vi "83-86 (SubVI).vi"(1 "String":string) -> (0 "Output":T1)   [LabVIEW 2024]
panel:
  in  "Output 2":T1
  in  "Carrier Card Temperature alert 2":T2
  in  "Switching Card 5 Temperature alert 2":T3
  in  "Switching Card 4 Temperature alert 2":T4
  in  "Switching Card 3 Temperature alert 2":T5
  in  "Switching Card 2 Temperature alert 2":T6
  in  "Switching Card 1 Temperature alert  2":T7
  in  "Control Card Temperature alert  2":T8
  in  "Carrier Card Temperature Warning 2":T9
  in  "Switching Card 5 Temperature Warning 2":T10
  in  "Switching Card 4 Temperature  Warning 2":T11
  in  "Switching Card 3 Temperature Warning 2":T12
  in  "Switching Card 2 Temperature High Warning 2":T13
  in  "Switching Card 1 Temperature Warning 2":T14
  in  "Control Card Temperature Warning 2":T15
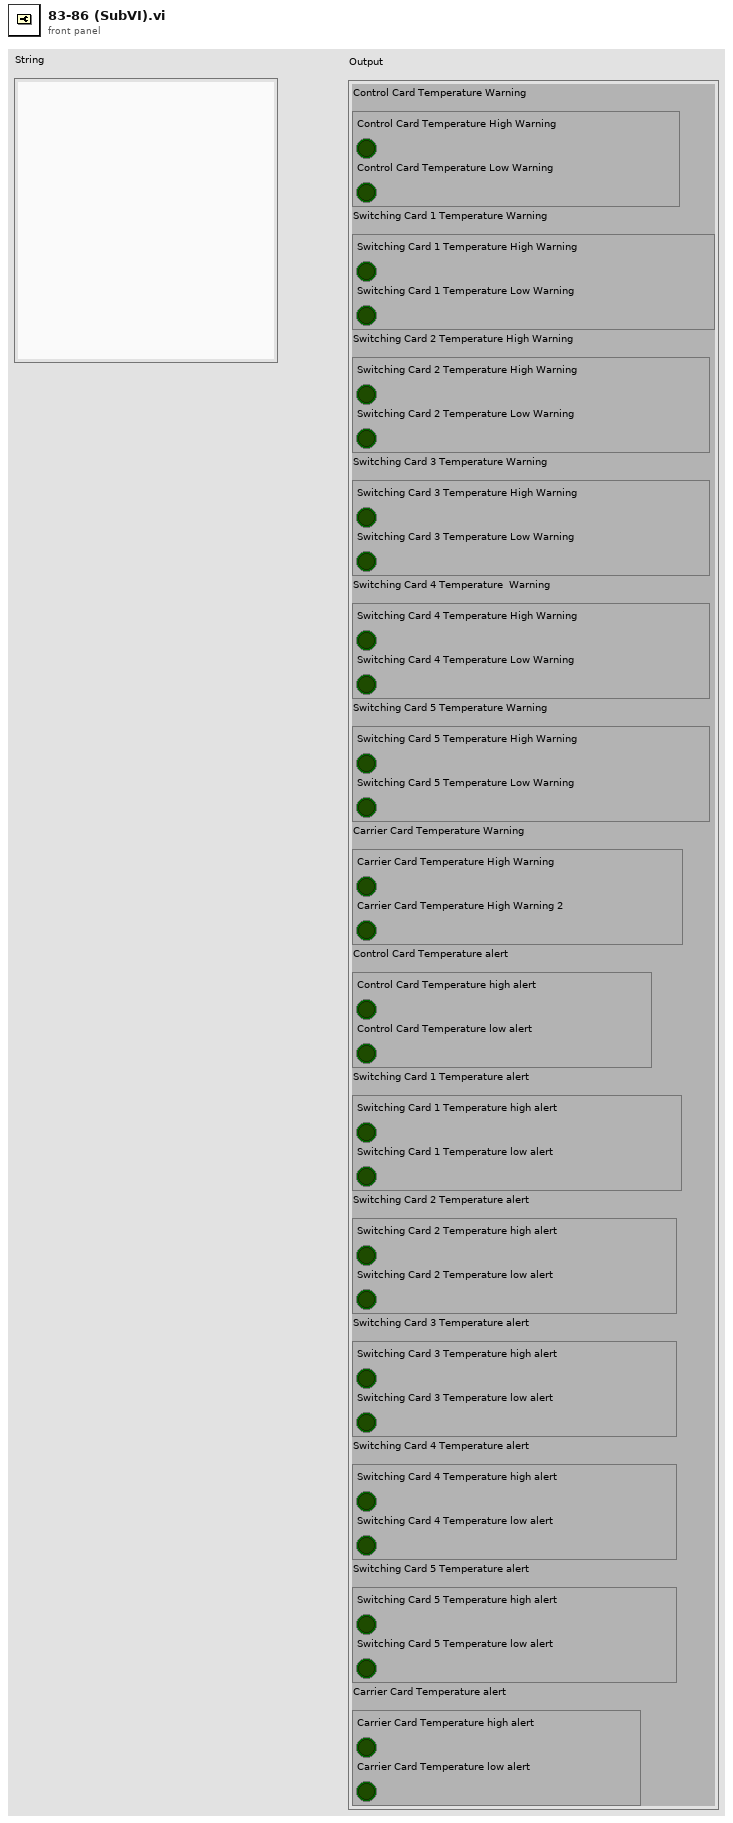
[diagram p1: front panel]
types:
  T1 = cluster{"Control Card Temperature Warning":cluster{"Control Card Temperature High Warning ":bool, "Control Card Temperature Low Warning":bool}, "Switching Card 1 Temperature Warning":cluster{"Switching Card 1 Temperature High Warning ":bool, "Switching Card 1 Temperature Low Warning":bool}, "Switching Card 2 Temperature High Warning":cluster{"Switching Card 2 Temperature High Warning":bool, "Switching Card 2 Temperature Low Warning":bool}, "Switching Card 3 Temperature Warning":cluster{"Switching Card 3 Temperature High Warning":bool, "Switching Card 3 Temperature Low Warning":bool}, "Switching Card 4 Temperature  Warning":cluster{"Switching Card 4 Temperature High Warning":bool, "Switching Card 4 Temperature Low Warning":bool}, "Switching Card 5 Temperature Warning":cluster{"Switching Card 5 Temperature High Warning":bool, "Switching Card 5 Temperature Low Warning":bool}, "Carrier Card Temperature Warning":cluster{"Carrier Card Temperature High Warning":bool, "Carrier Card Temperature High Warning 2":bool}, "Control Card Temperature alert ":cluster{"Control Card Temperature high alert ":bool, "Control Card Temperature low alert ":bool}, "Switching Card 1 Temperature alert ":cluster{"Switching Card 1 Temperature high alert ":bool, "Switching Card 1 Temperature low alert ":bool}, "Switching Card 2 Temperature alert":cluster{"Switching Card 2 Temperature high alert":bool, "Switching Card 2 Temperature low alert":bool}, "Switching Card 3 Temperature alert":cluster{"Switching Card 3 Temperature high alert":bool, "Switching Card 3 Temperature low alert":bool}, "Switching Card 4 Temperature alert":cluster{"Switching Card 4 Temperature high alert":bool, "Switching Card 4 Temperature low alert":bool}, "Switching Card 5 Temperature alert":cluster{"Switching Card 5 Temperature high alert":bool, "Switching Card 5 Temperature low alert":bool}, "Carrier Card Temperature alert":cluster{"Carrier Card Temperature high alert":bool, "Carrier Card Temperature low alert":bool}}
  T2 = cluster{"Carrier Card Temperature high alert":bool, "Carrier Card Temperature low alert":bool}
  T3 = cluster{"Switching Card 5 Temperature high alert":bool, "Switching Card 5 Temperature low alert":bool}
  T4 = cluster{"Switching Card 4 Temperature high alert":bool, "Switching Card 4 Temperature low alert":bool}
  T5 = cluster{"Switching Card 3 Temperature high alert":bool, "Switching Card 3 Temperature low alert":bool}
  T6 = cluster{"Switching Card 2 Temperature high alert":bool, "Switching Card 2 Temperature low alert":bool}
  T7 = cluster{"Switching Card 1 Temperature high alert ":bool, "Switching Card 1 Temperature low alert ":bool}
  T8 = cluster{"Control Card Temperature high alert ":bool, "Control Card Temperature low alert ":bool}
  T9 = cluster{"Carrier Card Temperature High Warning":bool, "Carrier Card Temperature High Warning 2":bool}
  T10 = cluster{"Switching Card 5 Temperature High Warning":bool, "Switching Card 5 Temperature Low Warning":bool}
  T11 = cluster{"Switching Card 4 Temperature High Warning":bool, "Switching Card 4 Temperature Low Warning":bool}
  T12 = cluster{"Switching Card 3 Temperature High Warning":bool, "Switching Card 3 Temperature Low Warning":bool}
  T13 = cluster{"Switching Card 2 Temperature High Warning":bool, "Switching Card 2 Temperature Low Warning":bool}
  T14 = cluster{"Switching Card 1 Temperature High Warning ":bool, "Switching Card 1 Temperature Low Warning":bool}
  T15 = cluster{"Control Card Temperature High Warning ":bool, "Control Card Temperature Low Warning":bool}
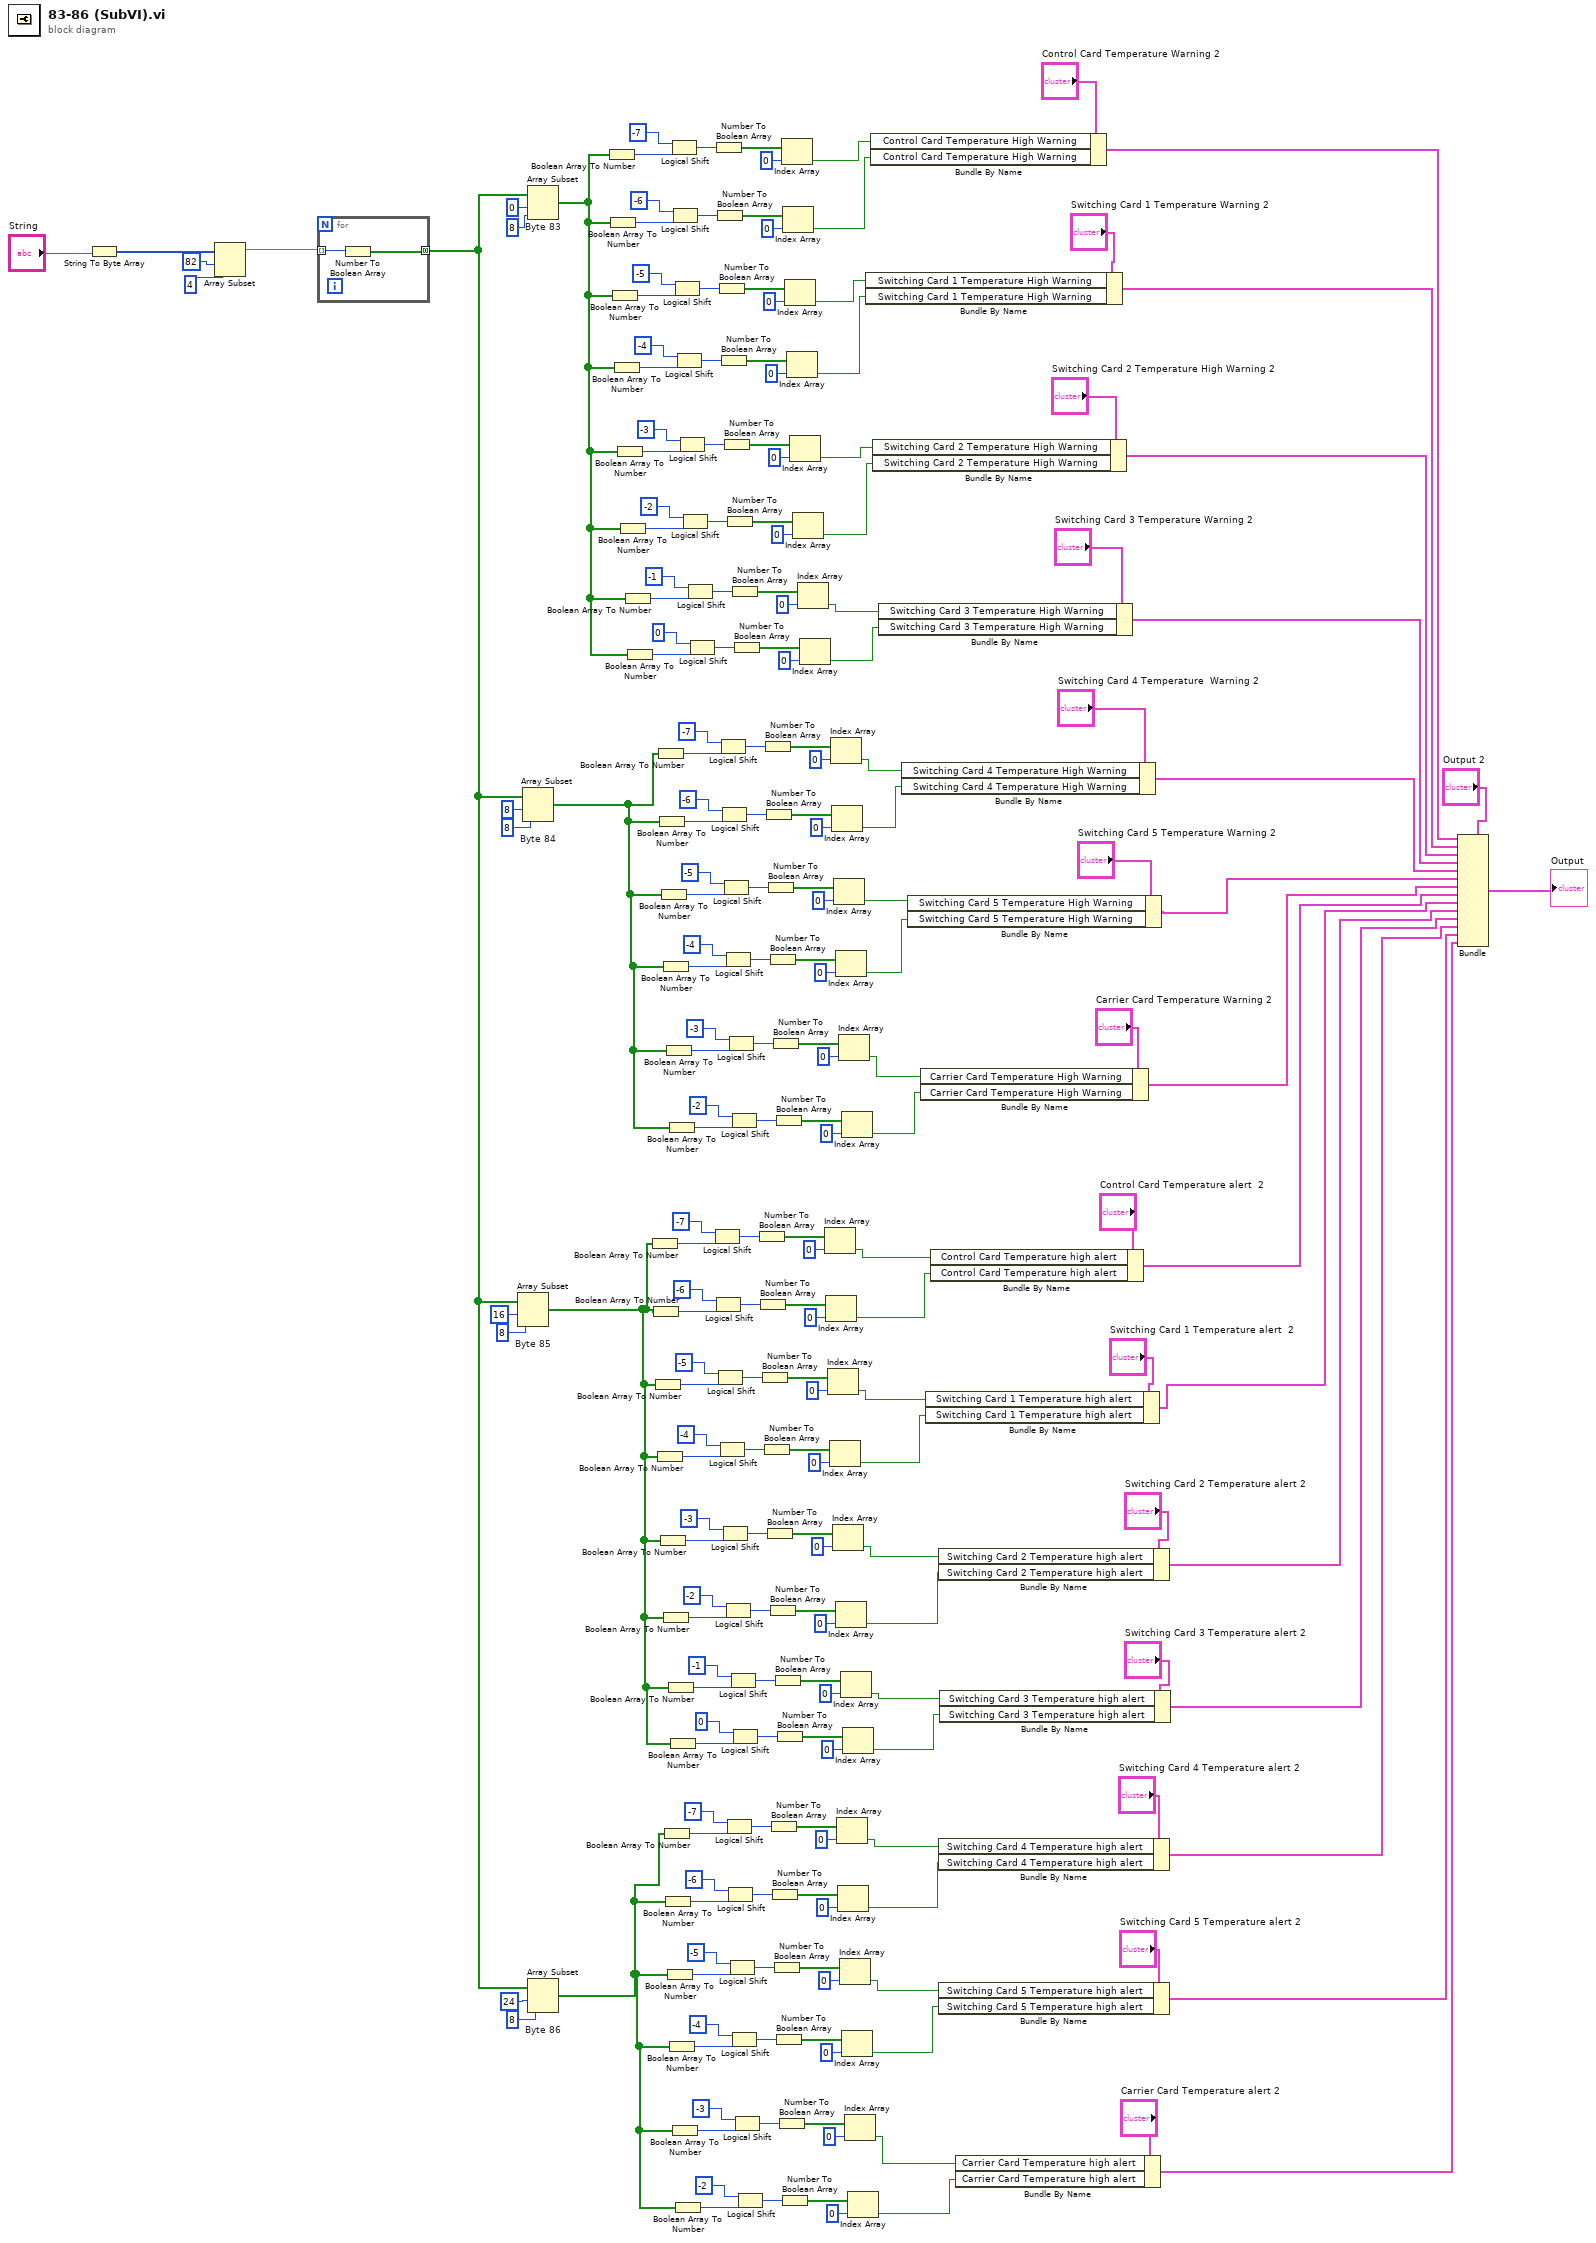
[diagram p0: block diagram]
diagram:
  n1 = String To Byte Array(string="String") -> (unsigned byte array=w209:u8[])
  n2 = Array Subset(array=w209, index=82, length=4) -> (w206:u8[])
  n3 = for {
    tunnel: w206 -> [w218] mode=indexing
    tunnel: [w217] -> w203 mode=concatenating
    n4 = Number To Boolean Array(number=w218) -> (Boolean array=w217:bool[])
  }
  n5 = Array Subset "Byte 85"(array=w203, index=16, length=8) -> (w90:bool[])
  n6 = Array Subset "Byte 84"(array=w203, index=8, length=8) -> (w131:bool[])
  n7 = Array Subset "Byte 83"(array=w203, index=0, length=8) -> (w162:bool[])
  n8 = Array Subset "Byte 86"(array=w203, index=24, length=8) -> (w59:bool[])
  n9 = Boolean Array To Number(Boolean array=w162) -> (number=w200:u32)
  n10 = Boolean Array To Number(Boolean array=w162) -> (number=w195:u32)
  n11 = Boolean Array To Number(Boolean array=w162) -> (number=w190:u32)
  n12 = Boolean Array To Number(Boolean array=w162) -> (number=w185:u32)
  n13 = Boolean Array To Number(Boolean array=w162) -> (number=w180:u32)
  n14 = Boolean Array To Number(Boolean array=w162) -> (number=w175:u32)
  n15 = Boolean Array To Number(Boolean array=w162) -> (number=w170:u32)
  n16 = Boolean Array To Number(Boolean array=w162) -> (number=w165:u32)
  n17 = Boolean Array To Number(Boolean array=w90) -> (number=w93:u32)
  n18 = Boolean Array To Number(Boolean array=w90) -> (number=w98:u32)
  n19 = Boolean Array To Number(Boolean array=w90) -> (number=w103:u32)
  n20 = Boolean Array To Number(Boolean array=w90) -> (number=w108:u32)
  n21 = Boolean Array To Number(Boolean array=w131) -> (number=w134:u32)
  n22 = Boolean Array To Number(Boolean array=w131) -> (number=w139:u32)
  n23 = Boolean Array To Number(Boolean array=w90) -> (number=w113:u32)
  n24 = Boolean Array To Number(Boolean array=w131) -> (number=w144:u32)
  n25 = Boolean Array To Number(Boolean array=w131) -> (number=w149:u32)
  n26 = Boolean Array To Number(Boolean array=w90) -> (number=w118:u32)
  n27 = Boolean Array To Number(Boolean array=w59) -> (number=w87:u32)
  n28 = Boolean Array To Number(Boolean array=w59) -> (number=w82:u32)
  n29 = Boolean Array To Number(Boolean array=w131) -> (number=w154:u32)
  n30 = Boolean Array To Number(Boolean array=w59) -> (number=w77:u32)
  n31 = Boolean Array To Number(Boolean array=w90) -> (number=w123:u32)
  n32 = Boolean Array To Number(Boolean array=w131) -> (number=w159:u32)
  n33 = Boolean Array To Number(Boolean array=w59) -> (number=w72:u32)
  n34 = Boolean Array To Number(Boolean array=w90) -> (number=w128:u32)
  n35 = Logical Shift(y=i16 -7, x=w200) -> (x << y=w202:u32)
  n36 = Logical Shift(y=i16 -6, x=w195) -> (x << y=w193:u32)
  n37 = Boolean Array To Number(Boolean array=w59) -> (number=w67:u32)
  n38 = Logical Shift(y=i16 -5, x=w190) -> (x << y=w192:u32)
  n39 = Boolean Array To Number(Boolean array=w59) -> (number=w62:u32)
  n40 = Logical Shift(y=i16 -4, x=w185) -> (x << y=w183:u32)
  n41 = Logical Shift(y=i16 -3, x=w180) -> (x << y=w182:u32)
  n42 = Logical Shift(y=i16 -2, x=w175) -> (x << y=w173:u32)
  n43 = Logical Shift(y=i16 -1, x=w170) -> (x << y=w172:u32)
  n44 = Logical Shift(y=i16 0, x=w165) -> (x << y=w163:u32)
  n45 = Logical Shift(y=i16 -7, x=w93) -> (x << y=w91:u32)
  n46 = Logical Shift(y=i16 -6, x=w98) -> (x << y=w100:u32)
  n47 = Number To Boolean Array(number=w202) -> (Boolean array=w199:bool[])
  n48 = Number To Boolean Array(number=w193) -> (Boolean array=w196:bool[])
  n49 = Logical Shift(y=i16 -5, x=w103) -> (x << y=w101:u32)
  n50 = Number To Boolean Array(number=w192) -> (Boolean array=w189:bool[])
  n51 = Logical Shift(y=i16 -4, x=w108) -> (x << y=w110:u32)
  n52 = Logical Shift(y=i16 -7, x=w134) -> (x << y=w132:u32)
  n53 = Number To Boolean Array(number=w183) -> (Boolean array=w186:bool[])
  n54 = Logical Shift(y=i16 -6, x=w139) -> (x << y=w141:u32)
  n55 = Logical Shift(y=i16 -3, x=w113) -> (x << y=w111:u32)
  n56 = Logical Shift(y=i16 -5, x=w144) -> (x << y=w142:u32)
  n57 = Number To Boolean Array(number=w182) -> (Boolean array=w179:bool[])
  n58 = Logical Shift(y=i16 -4, x=w149) -> (x << y=w151:u32)
  n59 = Logical Shift(y=i16 -2, x=w118) -> (x << y=w120:u32)
  n60 = Logical Shift(y=i16 -7, x=w87) -> (x << y=w89:u32)
  n61 = Number To Boolean Array(number=w173) -> (Boolean array=w176:bool[])
  n62 = Logical Shift(y=i16 -6, x=w82) -> (x << y=w80:u32)
  n63 = Logical Shift(y=i16 -3, x=w154) -> (x << y=w152:u32)
  n64 = Logical Shift(y=i16 -5, x=w77) -> (x << y=w79:u32)
  n65 = Logical Shift(y=i16 -1, x=w123) -> (x << y=w121:u32)
  n66 = Logical Shift(y=i16 -2, x=w159) -> (x << y=w161:u32)
  n67 = Logical Shift(y=i16 -4, x=w72) -> (x << y=w70:u32)
  n68 = Number To Boolean Array(number=w172) -> (Boolean array=w169:bool[])
  n69 = Logical Shift(y=i16 0, x=w128) -> (x << y=w130:u32)
  n70 = Number To Boolean Array(number=w163) -> (Boolean array=w166:bool[])
  n71 = Logical Shift(y=i16 -3, x=w67) -> (x << y=w69:u32)
  n72 = Logical Shift(y=i16 -2, x=w62) -> (x << y=w60:u32)
  n73 = Number To Boolean Array(number=w91) -> (Boolean array=w94:bool[])
  n74 = Number To Boolean Array(number=w100) -> (Boolean array=w97:bool[])
  n75 = Number To Boolean Array(number=w101) -> (Boolean array=w104:bool[])
  n76 = Number To Boolean Array(number=w110) -> (Boolean array=w107:bool[])
  n77 = Number To Boolean Array(number=w132) -> (Boolean array=w135:bool[])
  n78 = Number To Boolean Array(number=w141) -> (Boolean array=w138:bool[])
  n79 = Number To Boolean Array(number=w111) -> (Boolean array=w114:bool[])
  n80 = Number To Boolean Array(number=w142) -> (Boolean array=w145:bool[])
  n81 = Number To Boolean Array(number=w151) -> (Boolean array=w148:bool[])
  n82 = Number To Boolean Array(number=w120) -> (Boolean array=w117:bool[])
  n83 = Number To Boolean Array(number=w89) -> (Boolean array=w86:bool[])
  n84 = Number To Boolean Array(number=w80) -> (Boolean array=w83:bool[])
  n85 = Number To Boolean Array(number=w152) -> (Boolean array=w155:bool[])
  n86 = Number To Boolean Array(number=w79) -> (Boolean array=w76:bool[])
  n87 = Number To Boolean Array(number=w121) -> (Boolean array=w124:bool[])
  n88 = Number To Boolean Array(number=w161) -> (Boolean array=w158:bool[])
  n89 = Number To Boolean Array(number=w70) -> (Boolean array=w73:bool[])
  n90 = Number To Boolean Array(number=w130) -> (Boolean array=w127:bool[])
  n91 = Number To Boolean Array(number=w69) -> (Boolean array=w66:bool[])
  n92 = Number To Boolean Array(number=w60) -> (Boolean array=w63:bool[])
  n93 = Index Array(array=w199, index=0) -> (element=w28:bool)
  n94 = Index Array(array=w196, index=0) -> (element=w27:bool)
  n95 = Index Array(array=w189, index=0) -> (element=w26:bool)
  n96 = Index Array(array=w186, index=0) -> (element=w25:bool)
  n97 = Index Array(array=w179, index=0) -> (element=w24:bool)
  n98 = Index Array(array=w176, index=0) -> (element=w23:bool)
  n99 = Index Array(array=w169, index=0) -> (element=w22:bool)
  n100 = Index Array(array=w166, index=0) -> (element=w21:bool)
  n101 = Index Array(array=w94, index=0) -> (element=w14:bool)
  n102 = Index Array(array=w97, index=0) -> (element=w13:bool)
  n103 = Index Array(array=w104, index=0) -> (element=w12:bool)
  n104 = Index Array(array=w107, index=0) -> (element=w11:bool)
  n105 = Index Array(array=w135, index=0) -> (element=w20:bool)
  n106 = Index Array(array=w138, index=0) -> (element=w19:bool)
  n107 = Index Array(array=w114, index=0) -> (element=w10:bool)
  n108 = Index Array(array=w145, index=0) -> (element=w18:bool)
  n109 = Index Array(array=w148, index=0) -> (element=w17:bool)
  n110 = Index Array(array=w117, index=0) -> (element=w9:bool)
  n111 = Index Array(array=w86, index=0) -> (element=w6:bool)
  n112 = Index Array(array=w83, index=0) -> (element=w5:bool)
  n113 = Index Array(array=w155, index=0) -> (element=w16:bool)
  n114 = Index Array(array=w76, index=0) -> (element=w4:bool)
  n115 = Index Array(array=w124, index=0) -> (element=w8:bool)
  n116 = Index Array(array=w158, index=0) -> (element=w15:bool)
  n117 = Index Array(array=w73, index=0) -> (element=w3:bool)
  n118 = Index Array(array=w127, index=0) -> (element=w7:bool)
  n119 = Index Array(array=w66, index=0) -> (element=w2:bool)
  n120 = Index Array(array=w63, index=0) -> (element=w1:bool)
  n121 = Bundle By Name(cluster="Switching Card 1 Temperature Warning 2", "Switching Card 1 Temperature High Warning"=w26, "Switching Card 1 Temperature High Warning"=w25) -> (w42:T14)
  n122 = Bundle By Name(cluster="Control Card Temperature Warning 2", "Control Card Temperature High Warning"=w28, "Control Card Temperature High Warning"=w27) -> (w43:T15)
  n123 = Bundle By Name(cluster="Switching Card 2 Temperature High Warning 2", "Switching Card 2 Temperature High Warning"=w24, "Switching Card 2 Temperature High Warning"=w23) -> (w41:T13)
  n124 = Bundle By Name(cluster="Switching Card 3 Temperature Warning 2", "Switching Card 3 Temperature High Warning"=w22, "Switching Card 3 Temperature High Warning"=w21) -> (w40:T12)
  n125 = Bundle By Name(cluster="Switching Card 4 Temperature  Warning 2", "Switching Card 4 Temperature High Warning"=w20, "Switching Card 4 Temperature High Warning"=w19) -> (w39:T11)
  n126 = Bundle By Name(cluster="Switching Card 5 Temperature Warning 2", "Switching Card 5 Temperature High Warning"=w18, "Switching Card 5 Temperature High Warning"=w17) -> (w38:T10)
  n127 = Bundle By Name(cluster="Carrier Card Temperature Warning 2", "Carrier Card Temperature High Warning"=w16, "Carrier Card Temperature High Warning"=w15) -> (w37:T9)
  n128 = Bundle By Name(cluster="Switching Card 1 Temperature alert  2", "Switching Card 1 Temperature high alert"=w12, "Switching Card 1 Temperature high alert"=w11) -> (w35:T7)
  n129 = Bundle By Name(cluster="Control Card Temperature alert  2", "Control Card Temperature high alert"=w14, "Control Card Temperature high alert"=w13) -> (w36:T8)
  n130 = Bundle By Name(cluster="Switching Card 2 Temperature alert 2", "Switching Card 2 Temperature high alert"=w10, "Switching Card 2 Temperature high alert"=w9) -> (w34:T6)
  n131 = Bundle By Name(cluster="Switching Card 4 Temperature alert 2", "Switching Card 4 Temperature high alert"=w6, "Switching Card 4 Temperature high alert"=w5) -> (w32:T4)
  n132 = Bundle By Name(cluster="Switching Card 5 Temperature alert 2", "Switching Card 5 Temperature high alert"=w4, "Switching Card 5 Temperature high alert"=w3) -> (w31:T3)
  n133 = Bundle By Name(cluster="Switching Card 3 Temperature alert 2", "Switching Card 3 Temperature high alert"=w8, "Switching Card 3 Temperature high alert"=w7) -> (w33:T5)
  n134 = Bundle By Name(cluster="Carrier Card Temperature alert 2", "Carrier Card Temperature high alert"=w2, "Carrier Card Temperature high alert"=w1) -> (w30:T2)
  n135 = Bundle(cluster="Output 2", "Control Card Temperature Warning"=w43, "Switching Card 1 Temperature Warning"=w42, "Switching Card 2 Temperature High Warning"=w41, "Switching Card 3 Temperature Warning"=w40, "Switching Card 4 Temperature  Warning"=w39, "Switching Card 5 Temperature Warning"=w38, "Carrier Card Temperature Warning"=w37, "Control Card Temperature alert"=w36, "Switching Card 1 Temperature alert"=w35, "Switching Card 2 Temperature alert"=w34, "Switching Card 3 Temperature alert"=w33, "Switching Card 4 Temperature alert"=w32, "Switching Card 5 Temperature alert"=w31, "Carrier Card Temperature alert"=w30) -> (→"Output":T1)
